vi "PH_Beckhoff_PP_Control.write Conductivity to PSDB.vi"(0 "i ref in":refnum<vi>, 5 "error IO":errorcluster) -> (14 "i ref out":refnum<vi>, 19 "error out":errorcluster)   [LabVIEW 2014, in "PH_Beckhoff_PP_Control.lvlib"]
doc: "This VI writes the conductivity data to the PHELIX shot data base."
uses:
  PH_Beckhoff_PP_Control.lvlib
  PH_StatusHandler/PH_StatusHandler.Status.ctl
  PH_PSDBWriter/PH_PSDBWriter.Data Status.ctl
  PH_Beckhoff/PH_Beckhoff.lvlib
  CSCore/CSSystem/CSSystemLib/CSSystemLib.lvlib
  PH_PSDBWriter/PH_PSDBWriter.lvlib
  PH_Common/PH_Common.lvlib
  PH_StatusHandler/PH_StatusHandler.lvlib
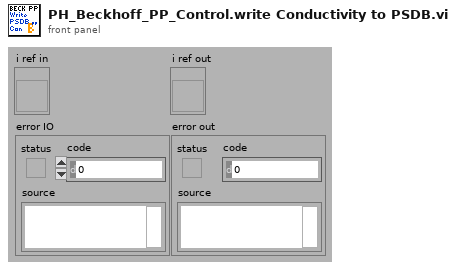
[diagram p1: front panel]
types:
  T1 = typedef "PH_Beckhoff.lvlib/PH_Beckhoff.i attribute.ctl" = cluster{"GUI Refs":T2, "operation?":bool, "Default Prdc Interval":i32, "Connection":T3, "AMS Net ID":T4, "Klemmencluster: # of":T5, "Values":T6, "IP":string, "Description":string, "configured?":bool, "Change Manager":cluster{"Detemination wanted?":bool, "Values changed at":cluster{"Sonderklemmen Inputs":i32[], "Analog Inputs":i32[], "Analog Outputs":i32[], "Digital Inputs":i32[], "Digital Outputs":i32[]}}, "Difference to handle an analog input as change":u32}
  T2 = typedef "PH_Beckhoff.lvlib/PH_Beckhoff.GUI Refs.ctl" = cluster{"ADS Error":refnum<vi>, "Values":refnum<vi>, "configured?":refnum<vi>, "Connection":refnum<vi>, "IP":refnum<vi>, "Prdc Int [ms]":refnum<vi>}
  T3 = typedef "PH_Beckhoff.lvlib/PH_Beckhoff.Connectivity.ctl" = cluster{"DLL?":bool, "Port?":bool, "Client?":bool, "Ping?":bool, "unsuccessful Pings":u32}
  T4 = typedef "Beckhoff - Driver np.lvlib/Beckhoff Access.ctl" = cluster{"DLL path":path, "AMS Net ID":cluster{"1st # of IP":u8, "2nd # of IP":u8, "3rd # of IP":u8, "4th # of IP":u8, "In Port":u8, "Out Port":u8}}
  T5 = typedef "Beckhoff - Driver np.lvlib/Klemmendeclarer.ctl" = cluster{"Offset due to Sonderklemms":u32, "analog Inputs":u32, "analog Outputs":u32, "digital Input Bits":u32, "digital Output Bits":u32}
  T6 = typedef "PH_Beckhoff.lvlib/PH_Beckhoff.Values.ctl" = cluster{"Sonderklemmen Inputs":T7, "Analog Inputs":T8, "Analog Outputs":T10, "Digital Inputs":T11, "Digital Outputs":T12}
  T7 = typedef "PH_Beckhoff.lvlib/PH_Beckhoff.Sonderklemmen Inputs.ctl" = cluster{"Total Length":u32, "Name":string, "Value":u64, "Quality":bool, "Service ID":i32, "Offset":u32, "Length":u32}[]
  T8 = typedef "PH_Beckhoff.lvlib/PH_Beckhoff.Analog Inputs.ctl" = cluster{"Name":string, "Value":u32, "Quality":bool, "Service ID":i32, "Sca Type":T9}[]
  T9 = typedef "PH_Beckhoff.lvlib/PH_Beckhoff.Scaling Type.ctl" = enum16{"none", "0 ... 15 Bit -> 0 ... 5", "0 ... 15 Bit -> 0 ... 10", "0 ... 15 Bit -> 0 ... 25", "0 ... 15 Bit -> 4 ... 20", "0 ... 15 Bit -> 0 ... 1", "0 ... 15 Bit -> 0 ... 20000", "0 ... 15 Bit -> 0 ... 24000"}
  T10 = typedef "PH_Beckhoff.lvlib/PH_Beckhoff.Analog Outputs.ctl" = cluster{"Name":string, "Value":u32, "Quality":bool, "Wanted Value":u32, "Service ID":i32, "Sca Type":T9}[]
  T11 = typedef "PH_Beckhoff.lvlib/PH_Beckhoff.Digital Inputs.ctl" = cluster{"Name":string, "Value":bool, "Quality":bool, "Service ID":i32, "inverted?":bool}[]
  T12 = typedef "PH_Beckhoff.lvlib/PH_Beckhoff.Digital Outputs.ctl" = cluster{"Name":string, "Value":bool, "Quality":bool, "Wanted Value":bool, "Service ID":i32, "inverted?":bool}[]
  T13 = typedef "PH_Beckhoff_PP_Control.lvlib/PH_Beckhoff_PP_Control.i attribute.ctl" = cluster{"PP Conductivity Control":cluster{"PSDB":cluster{"Status Service ID":i32, "Instance ID":i32, "Data Status":T14, "Ref Status":refnum<vi>, "Error Code":i32}, "Status":cluster{"GUI Ref":refnum<vi>, "Status Service ID":i32, "Status":T15}, "DIs":cluster{"Device on":cluster{"GUI Ref":refnum<vi>, "# in Data":i32}, "Conductivity ok":cluster{"GUI Ref":refnum<vi>, "# in Data":i32}, "Temperature ok":cluster{"GUI Ref":refnum<vi>, "# in Data":i32}, "Alarm":cluster{"GUI Ref":refnum<vi>, "# in Data":i32}}, "PSDB Thread":cluster{"Ref":refnum<vi>, "Q-Ref":refnum<queue>}}, "PP Mercury Control":cluster{"PSDB":cluster{"Status Service ID":i32, "Instance ID":i32, "Data Status":T14, "Ref Status":refnum<vi>, "Error Code":i32}, "Status":cluster{"GUI Ref":refnum<vi>, "Status Service ID":i32, "Status":T15}, "on since:":cluster{"GUI Ref":refnum<vi>, "Service ID":i32, "Time":string}, "DIs":cluster{"Device on":cluster{"GUI Ref":refnum<vi>, "# in Data":i32}, "Alarm":cluster{"GUI Ref":refnum<vi>, "# in Data":i32}}, "AIs":cluster{"Concentration":cluster{"GUI Ref":refnum<vi>, "# in Data":i32}}, "PSDB Thread":cluster{"Ref":refnum<vi>, "Q-Ref":refnum<queue>}}, "PSDB":cluster{"Shot #":i32, "Subsystem":T16}, "PSDB Credentials":T17}
  T14 = typedef "PH_PSDBWriter.lvlib/PH_PSDBWriter.Data Status.ctl" = i16
  T15 = typedef "PH_StatusHandler.lvlib/PH_StatusHandler.Status.ctl" = i16
  T16 = typedef "PH_PSDBWriter.lvlib/PH_PSDBWriter.PHELIX-Subsystems.ctl" = i32
  T17 = typedef "PH_Common.lvlib/PH_Connection.PSDB Credentials.ctl" = cluster{"PW":string, "ID":string, "DS":string}
  T18 = typedef "PH_PSDBWriter.lvlib/PH_PSDBWriter.String dataset.ctl" = cluster{"name":string, "data":string, "unit":string}
  T19 = typedef "PH_PSDBWriter.lvlib/PH_PSDBWriter.PSDB Dataset.ctl" = cluster{"Version":i32, "2D data Input":T20[], "Boolean Input":T22[], "Image Input":T23[], "Numeric Input":T25[], "String Input":T18[]}
  T20 = typedef "PH_PSDBWriter.lvlib/PH_PSDBWriter.2D dataset.ctl" = cluster{"name":string, "data":dbl[][], "axis description":T21}
  T21 = typedef "PSDB.lvlib/PSDB_AxisDescription.ctl" = cluster{"x axis label":string, "y axis label":string, "x axis unit":string, "y axis unit":string}
  T22 = typedef "PH_PSDBWriter.lvlib/PH_PSDBWriter.Boolean dataset.ctl" = cluster{"name":string, "data":bool, "unit":string}
  T23 = typedef "PH_PSDBWriter.lvlib/PH_PSDBWriter.Image dataset.ctl" = cluster{"name":string, "data":T24, "unit":string}
  T24 = typedef "IMAQ Image.ctl" = refnum<image>
  T25 = typedef "PH_PSDBWriter.lvlib/PH_PSDBWriter.Numeric dataset.ctl" = cluster{"name":string, "data":dbl, "unit":string}
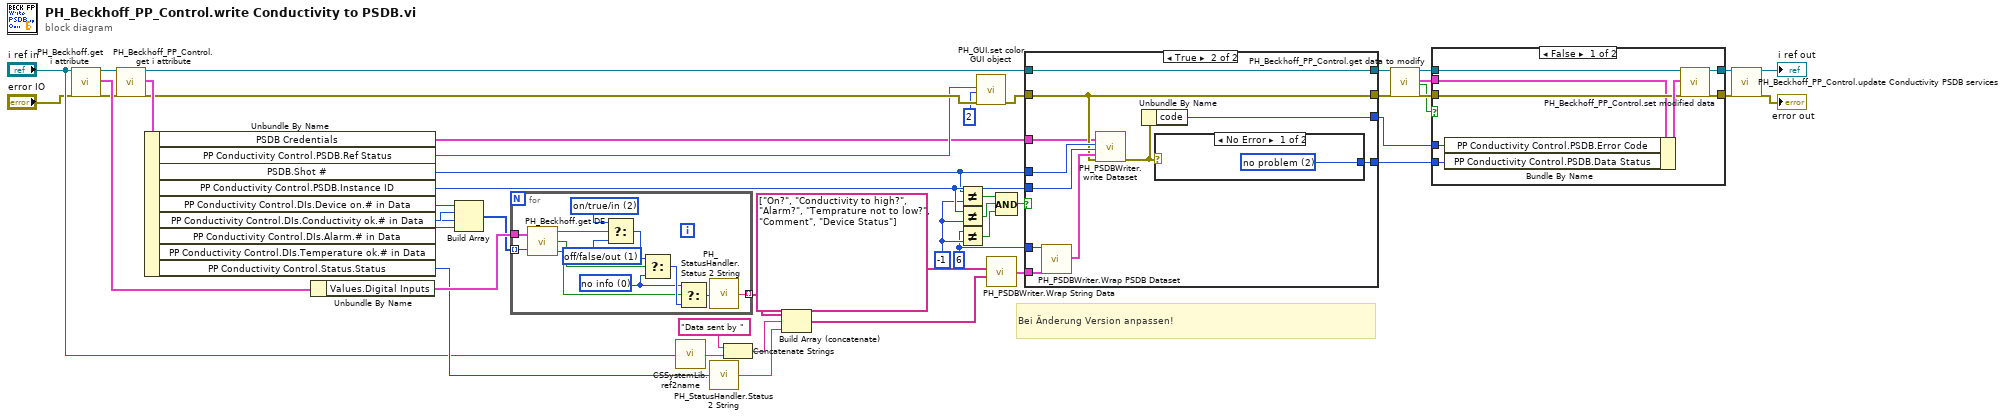
[diagram p0: block diagram]
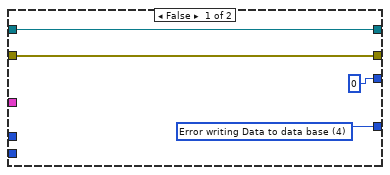
[diagram p3: hidden frame]
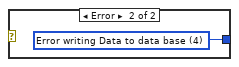
[diagram p4: hidden frame]
diagram:
  w34 = 6 ("Version")
  w40 = -1 ("y")
  # "Bei Änderung Version anpassen!"
  n1 = call "PH_Beckhoff.get i attribute.vi"("i ref in"="i ref in", "error in (no error)"="error IO") -> ("i ref out"=w12:refnum<vi>, "i attribute"=w21:T1, "error out"=w11:errorcluster)  [unwired: 15 in]
  n2 = call "PH_Beckhoff_PP_Control.get i attribute.vi"("i ref in"=w12, "error in (no error)"=w11) -> ("i ref out"=w9:refnum<vi>, "i attribute"=w10:T13, "error out"=w8:errorcluster)  [unwired: 15 in]
  n3 = Unbundle By Name(w10) -> ("PSDB Credentials"=w1:T17, "PP Conductivity Control.PSDB.Ref Status"=w6:refnum<vi>, "PSDB.Shot #"=w42:i32, "PP Conductivity Control.PSDB.Instance ID"=w43:i32, "PP Conductivity Control.DIs.Device on.# in Data"=w33:i32, "PP Conductivity Control.DIs.Conductivity ok.# in Data"=w32:i32, "PP Conductivity Control.DIs.Alarm.# in Data"=w31:i32, "PP Conductivity Control.DIs.Temperature ok.# in Data"=w30:i32, "PP Conductivity Control.Status.Status"=w22:T15)
  n4 = Unbundle By Name(w21) -> ("Values.Digital Inputs"=w29:T11)
  n5 = Build Array(w33, w32, w31, w30) -> (w28:i32[])
  n6 = for {
    tunnel: [w53] -> w27 mode=indexing
    tunnel: w29 -> [w49]
    tunnel: w28 -> [w48] mode=indexing
    w55 = T15 1 items=["no info", "off/false/out", "on/true/in", "Failure", "Alarm", "Status 1", "Status 2", "Status 3"] ("State Temp not 2 low")
    w56 = T15 2 items=["no info", "off/false/out", "on/true/in", "Failure", "Alarm", "Status 1", "Status 2", "Status 3"] ("State Temp not 2 low")
    w58 = T15 0 items=["no info", "off/false/out", "on/true/in", "Failure", "Alarm", "Status 1", "Status 2", "Status 3"] ("State Temp not 2 low")
    n7 = call "PH_Beckhoff.get DE.vi"("Digital Values"=w49, "index of element"=w48) -> ("Value"=w52:bool, "Quality"=w51:bool, "Tag not found"=w50:bool)
    n8 = Select(t=w56, s=w52, f=w55) -> (s? t:f=w57:T15)
    n9 = Select(t=w57, s=w51, f=w58) -> (s? t:f=w59:T15)
    n10 = Select(t=w58, s=w50, f=w59) -> (s? t:f=w54:T15)
    n11 = call "PH_StatusHandler.Status 2 String.vi"("Status"=w54) -> ("Status as string"=w53:string)
  }
  n12 = call "CSSystemLib.ref2name.vi"("obj refnum"="i ref in") -> ("name"=w25:string)
  n13 = call "PH_StatusHandler.Status 2 String.vi"("Status"=w22) -> ("Status as string"=w23:string)
  n14 = Concatenate Strings("Data sent by " ("string"), w25) -> (w24:string)
  n15 = Build Array (concatenate)(w27, w24, w23) -> (w3:string[])
  n16 = Not Equal?(x=w42, y=w40) -> (x != y?=w39:bool)
  n17 = Not Equal?(x=w43, y=w40) -> (x != y?=w38:bool)
  n18 = Not Equal?(x=w34, y=w40) -> (x != y?=w37:bool)
  n19 = call "PH_GUI.set color GUI object.vi"("GUI object Ref"=w6, "State"=2, "error in (no error)"=w8) -> ("error out"=w7:errorcluster)  [unwired: 16 in]
  n20 = call "PH_PSDBWriter.Wrap String Data.vi"("Data Array"=w3, "Name Array"=string[] ["On?", "Conductivity to high?", "Alarm?", "Temprature not to low?", "Comment", "Device Status"]) -> ("PSDB String Data Array"=w2:T18[])  [unwired: 2 in]
  n21 = Compound Arithmetic op=AND(w39, w38, w37) -> (w36:bool)
  n22 = case shown="True" w36 {
    tunnel: w7 -> [w61 w66]
    tunnel: w43 -> [_ w70]
    tunnel: w34 -> [_ w68]
    tunnel: [w63 w74] -> w41
    tunnel: w9 -> [w62 w73]
    tunnel: [w62 w73] -> w19
    tunnel: [w61 w66] -> w17
    tunnel: w42 -> [_ w71]
    tunnel: [0 ("code") w72] -> w35
    tunnel: w2 -> [_ w69]
    tunnel: w1 -> [_ w64]
    frame False {
      w63 = T14 4 items=["no info", "no Data collection", "no problem", "Error getting the instance ID", "Error writing Data to data base", "Error concerning the subsystem"] ("Data Status")
    }
    frame True {
      n23 = call "PH_PSDBWriter.Wrap PSDB Dataset.vi"("Version"=w68, "String Input"=w69) -> ("PSDB Dataset"=w67:T19)  [unwired: 17 in]
      n24 = call "PH_PSDBWriter.write Dataset.vi"("PSDB Credentials"=w64, "Shot #"=w71, "Instance ID"=w70, "Data to write to PSDB"=w67, "error in (no error)"=w66) -> ("error out"=w65:errorcluster)  [unwired: 14 in]
      n25 = Unbundle By Name(w65) -> ("code"=w72:i32)
      n26 = case shown="No Error" w65 {
        tunnel: [w75 w76] -> w74
        frame No Error {
          w75 = T14 2 items=["no info", "no Data collection", "no problem", "Error getting the instance ID", "Error writing Data to data base", "Error concerning the subsystem"] ("Data Status")
        }
        frame Error {
          w76 = T14 4 items=["no info", "no Data collection", "no problem", "Error getting the instance ID", "Error writing Data to data base", "Error concerning the subsystem"] ("Data Status")
        }
      }
    }
  }
  n27 = call "PH_Beckhoff_PP_Control.get data to modify.vi"("i ref in"=w19, "error in (no error)"=w17) -> ("i ref out"=w20:refnum<vi>, "i attribute"=w16:T13, "timed out"=w15:bool, "error out"=w18:errorcluster)  [unwired: 14 in]
  n28 = case shown="False" w15 {
    tunnel: [w84 w86] -> w45
    tunnel: [w83 w85] -> w47
    tunnel: w41 -> [w82 _]
    tunnel: w35 -> [w80 _]
    tunnel: w20 -> [w79 w86]
    tunnel: w18 -> [w78 w85]
    tunnel: w16 -> [w77 _]
    frame False {
      n29 = Bundle By Name(cluster=w77, "PP Conductivity Control.PSDB.Error Code"=w80, "PP Conductivity Control.PSDB.Data Status"=w82) -> (w81:T13)
      n30 = call "PH_Beckhoff_PP_Control.set modified data.vi"("i ref in"=w79, "i attribute"=w81, "error in (no error)"=w78) -> ("i ref out"=w84:refnum<vi>, "error out"=w83:errorcluster)  [unwired: 15 in]
    }
    frame True {
    }
  }
  n31 = call "PH_Beckhoff_PP_Control.update Conductivity PSDB services.vi"("i ref in"=w45, "error in"=w47) -> ("i ref out"=→"i ref out":refnum<vi>, "error out"=→"error out":errorcluster)  [unwired: 16 in]
